vi "Draw PIXY rects.vi"(8 "CC Objects":T1(array[cluster]), 9 "Draw Options":cluster{"Objects":bool, "CC Objects":bool}, 10 "Colors":u32[](array[colorbox]), 11 "Object":T2(array[cluster])) -> (3 "Picture":picture)   [LabVIEW 2016]
doc: "Draw the objects and color combo objects."
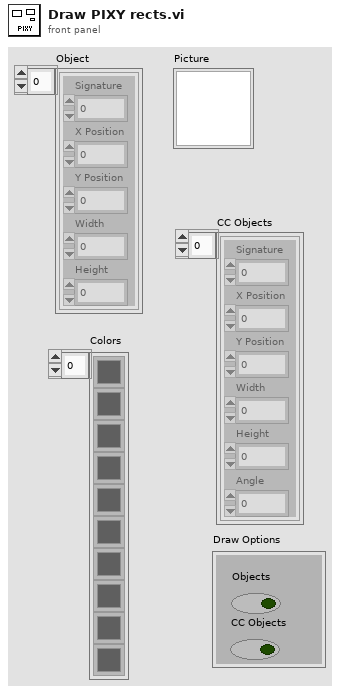
[diagram p1: front panel]
types:
  T1 = cluster{"Signature":u16, "X Position":u16, "Y Position":u16, "Width":u16, "Height":u16, "Angle":i16}[]
  T2 = cluster{"Signature":u16, "X Position":u16, "Y Position":u16, "Width":u16, "Height":u16}[]
  T3 = cluster{"X Position":u16, "Y Position":u16, u16, u16}
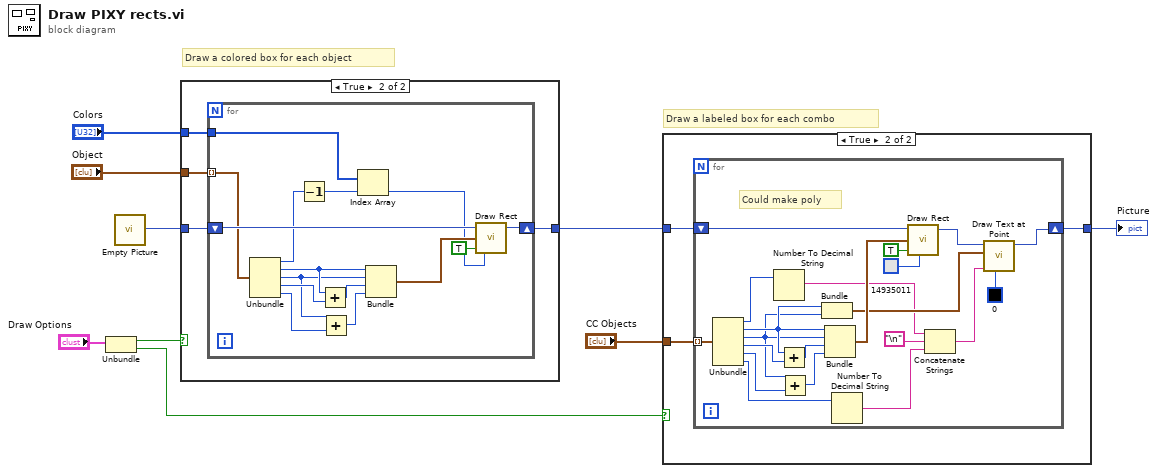
[diagram p0: block diagram]
diagram:
  # "Draw a labeled box for each combo"
  # "Draw a colored box for each object"
  n1 = Unbundle("Draw Options") -> ("Objects"=w4:bool, "CC Objects"=w2:bool)
  n2 = call "Empty Picture"() -> ("empty picture"=w8:picture)
  n3 = case shown="True" w4 {
    tunnel: "Object" -> [_ w14]
    tunnel: w8 -> [w10 w13]
    tunnel: "Colors" -> [_ w12]
    tunnel: [w10 w11] -> w6
    frame False {
    }
    frame True {
      n4 = for {
        tunnel: w14 -> [w28] mode=indexing
        shift-right: [w20] -> w11
        shift-left: w13 -> [w29]
        tunnel: w12 -> [w18]
        n5 = Unbundle(w28) -> ("Signature"=w19:u16, "X Position"=w27:u16, "Y Position"=w25:u16, "Width"=w26:u16, "Height"=w24:u16)
        n6 = Decrement(x=w19) -> (x-1=w17:u16)
        n7 = Add(x=w27, y=w26) -> (x+y=w23:u16)
        n8 = Add(x=w25, y=w24) -> (x+y=w22:u16)
        n9 = Index Array(array=w18, index=w17) -> (element=w16:u32)
        n10 = Bundle("X Position"=w27, "Y Position"=w25, w23, w22) -> (w21:T3)  [unwired: 1 in]
        n11 = call <vilib>:"Draw Rect.vi"("picture"=w29, "rect"=w21, "fill?(F)"=TRUE, "color(black)"=w16) -> ("new picture"=w20:picture)  [unwired: 5 in]
      }
    }
  }
  n12 = case shown="True" w2 {
    tunnel: w6 -> [w30 w33]
    tunnel: "CC Objects" -> [_ w32]
    tunnel: [w30 w31] -> w1
    frame False {
    }
    frame True {
      n13 = for {
        shift-right: [w44] -> w31
        shift-left: w33 -> [w52]
        tunnel: w32 -> [w54] mode=indexing
        # "Could make poly"
        n14 = Unbundle(w54) -> ("Signature"=w38:u16, "X Position"=w43:u16, "Y Position"=w42:u16, "Width"=w48:u16, "Height"=w47:u16, "Angle"=w40:i16)
        n15 = Number To Decimal String(number=w38) -> (decimal integer string=w37:string)  [unwired: 1 in]
        n16 = Add(x=w43, y=w48) -> (x+y=w50:u16)
        n17 = Add(x=w42, y=w47) -> (x+y=w51:u16)
        n18 = Bundle("X Position"=w43, "Y Position"=w42) -> (w41:cluster{"X Position":u16, "Y Position":u16})  [unwired: 1 in]
        n19 = Bundle("X Position"=w43, "Y Position"=w42, w50, w51) -> (w49:T3)  [unwired: 1 in]
        n20 = Number To Decimal String(number=w40) -> (decimal integer string=w35:string)  [unwired: 1 in]
        n21 = call <vilib>:"Draw Rect.vi"("picture"=w52, "rect"=w49, "fill?(F)"=TRUE, "color(black)"=u32 14935011) -> ("new picture"=w45:picture)  [unwired: 5 in]
        n22 = Concatenate Strings(w37, "\n", w35) -> (w36:string)
        n23 = call <vilib>:"Draw Text at Point.vi"("text color(black)"=u32 0, "text"=w36, "origin"=w41, "picture"=w45) -> ("new picture"=w44:picture)  [unwired: 6 in, 1 out]
      }
    }
  }
  "Picture" <- w1
